vi "PLC Test.vi"   [LabVIEW 2020]
uses:
  EventLogger.lvlibp/1abvi3w/vi.lib/gpm_packages/@cs/event-logger/Source/Composed Log/Types/Log Level.ctl
  EventLogger.lvlibp/1abvi3w/vi.lib/gpm_packages/@cs/event-logger/Source/Text File Sink/Configuration.ctl
  Abstract PLC Controler/Abstract PLC Controler.lvclass/Abstract PLC Controler.ctl
  InovanceSerial/InovanceSerial.lvclass
  D:/Git/Labview-Libraries/Libraries/HslCommunication/Abstract PLC Controler/Abstract PLC Controler.lvclass
  InovanceTCP/InovanceTCP.lvclass
  Abstract PLC Controler/Abstract PLC Controler.lvclass
  EventLogger.lvlibp/Logger.lvclass
  EventLogger.lvlibp/1abvi3w/vi.lib/gpm_packages/@cs/event-logger/Source/Composed Log/Composed Log.lvlib
  EventLogger.lvlibp/1abvi3w/vi.lib/gpm_packages/@cs/event-logger/Source/Text File Sink/Text File Sink.lvclass
types:
  T1 = typedef "EventLogger.lvlibp/Text File Sink.lvclass/Configuration.ctl" = cluster{"Folder":path, "Name":string, "Extension":string, "Max Size (MB)":i64, "Timestamp Filename":bool}
  T2 = typedef "EventLogger.lvlibp/Composed Log.lvlib/Log Level.ctl" = enum16{"Debug", "Info", "Warning", "Error", "Critical"}
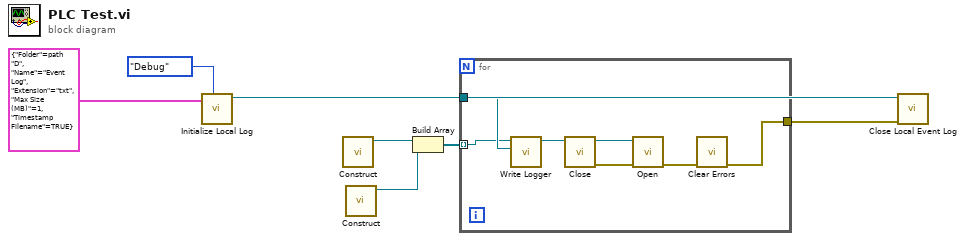
[diagram p0: block diagram]
diagram:
  n1 = call "Initialize Local Log.vi"("LogLevel"=Log_Level."Debug", "Text File Configuration"=T1 {"Folder"=path "D:/", "Name"="Event Log", "Extension"="txt", "Max Size (MB)"=1, "Timestamp Filename"=TRUE}) -> ("Logger out"=w5:refnum<class "Logger.lvclass">)  [unwired: 8 in, 1 out]
  n2 = call "Construct.vi"() -> ("MelsecMcNet out"=w1:refnum<class "InovanceSerial.lvclass">)  [unwired: 11 in]
  n3 = call "Construct.vi"() -> ("MelsecMcNet out"=w4:refnum<class "InovanceTCP.lvclass">)  [unwired: 11 in]
  n4 = Build Array(w1, w4) -> (w2:refnum<class "Abstract PLC Controler.lvclass">[])
  n5 = for {
    tunnel: w5 -> [w11]
    tunnel: [w9] -> w3
    tunnel: w2 -> [w8] mode=indexing
    n6 = call "Write Logger.vi"("EventLogger.lvlibp:Logger.lvclass"=w11, "Abstract PLC Controler in"=w8) -> ("Abstract PLC Controler out"=w14:refnum<class "Abstract PLC Controler.lvclass">)  [unwired: 9 in]
    n7 = call-dynamic "Close.vi"("MelsecTCP in"=w14) -> ("error out"=w12:errorcluster, "MelsecTCP out"=w13:refnum<class "Abstract PLC Controler.lvclass">)  [unwired: 9 in]
    n8 = call-dynamic "Open.vi"("error in (no error)"=w12, "MelsecTCP in"=w13) -> ("error out"=w10:errorcluster)  [unwired: 8 in, 1 out]
    n9 = call <vilib>:"Clear Errors.vi"("error in (no error)"=w10) -> ("error out"=w9:errorcluster)  [unwired: 5 in, 1 out]
  }
  n10 = call "Close Local Event Log.vi"("error in (no error)"=w3, "Logger in"=w5) -> ()  [unwired: 8 in, 2 out]
